vi "DecodeData.vi"(8 "error in (no error)":errorcluster, 9 "Secret":string, 10 "Encoded Data":string, 11 "CryptoType":refnum<class "Crypto.lvclass">) -> (0 "error out":errorcluster, 2 "Decoded Data":variant)   [LabVIEW 2016, in "Crypto.lvclass"]
uses:
  Crypto.lvclass
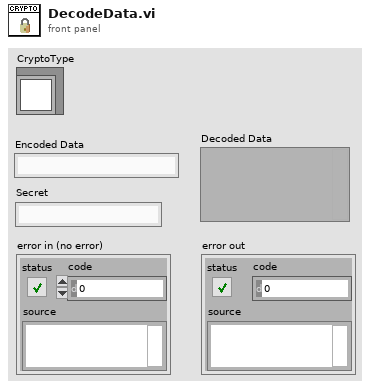
[diagram p1: front panel]
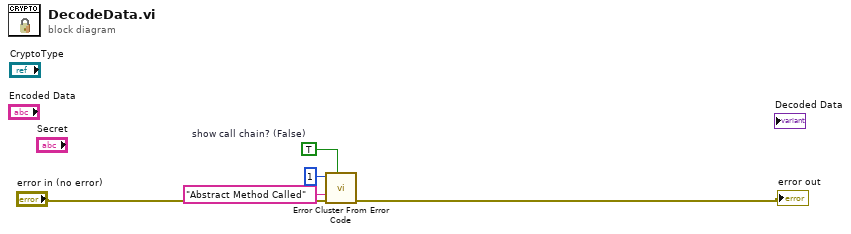
[diagram p0: block diagram]
diagram:
  w1 = TRUE  # show call chain? (False)
  n1 = call <vilib>:"Error Cluster From Error Code.vi"("show call chain? (False)"=w1, "error in (no error)"="error in (no error)", "error message (\"\")"="Abstract Method Called" ("error message (\"\")"), "error code (0)"=1) -> ("error out"=→"error out":errorcluster)  [unwired: 5 in]
